vi "VG_Ibms.vi"() -> ()   [LabVIEW 2020]
panel:
  out "VG_Ibms":dbl
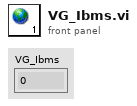
[diagram p1: front panel]
diagram:
